vi "NT1-Main.vi"() -> ()   [LabVIEW 2019]
uses:
  Get-Elapsed-Time.vi
  IsError.vi
  <vilib>/Rock Robotics/Network Tables/NT Globals.vi
  <vilib>/Rock Robotics/Network Tables/Manage Connection List.vi
  <vilib>/Rock Robotics/Network Tables/NT Write String Array.vi
  <vilib>/Rock Robotics/Network Tables/NT Write String.vi
  <vilib>/Rock Robotics/Network Tables/NT Write Numeric Array.vi
  <vilib>/Rock Robotics/Network Tables/NT Write Number.vi
  <vilib>/Rock Robotics/Network Tables/NT Write Boolean Array.vi
  <vilib>/Rock Robotics/Network Tables/NT Write Boolean.vi
  <vilib>/Rock Robotics/Network Tables/NT Read Boolean.vi
  <vilib>/Rock Robotics/Network Tables/NT Read Boolean Array.vi
  <vilib>/Rock Robotics/Network Tables/NT Read Number.vi
  <vilib>/Rock Robotics/Network Tables/NT Read Numeric Array.vi
  <vilib>/Rock Robotics/Network Tables/NT Read String.vi
  <vilib>/Rock Robotics/Network Tables/NT Read String Array.vi
  <vilib>/Rock Robotics/WPI/ThirdParty/JAS_Junk/TrajLib/Util_GetTime.vi
  NTJ_OldVer_FlushSingle.vi
  <vilib>/Rock Robotics/Network Tables/NT Flush Data Updates.vi
panel:
  out "Srv Test3 ID":i32 format="%11d"
  out "Srv Test2 ID":i32 format="%11d"
  out "Srv Test1 ID":i32 format="%11d"
  out "Srv Test0  ID":i32 format="%11d"
  out "Srv Test3 Seq":u16 format="0x%04x"
  out "Srv Test2 Seq":u16 format="0x%04x"
  out "Srv Test1 Seq":u16 format="0x%04x"
  out "Srv Test0  Seq":u16 format="0x%04x"
  out "Test3 ID":i32 format="%11d"
  out "Test2 ID":i32 format="%11d"
  out "Test1 ID":i32 format="%11d"
  out "Test0  ID":i32 format="%11d"
  out "Serv Test3":dbl
  out "Serv Test2":dbl
  out "ServTest1":dbl
  out "Serv Test0":dbl
  out "Serv Flush\nTest0":bool=TRUE
  out "Serv Set Fast":bool=TRUE
  out "Serv Create\nNew":bool=TRUE
  out "Serv Many Fast":bool=TRUE
  out "Serv Del New":bool=TRUE
  out "Serv Del All":bool=TRUE
  out "Serv Test1\nPersist":bool=TRUE
  out "Test1 \nPersist (flg)":bool=TRUE
  out "Test3 Seq":u16 format="0x%04x"
  out "Test2 Seq":u16 format="0x%04x"
  out "Test1 Seq":u16 format="0x%04x"
  out "Test0  Seq":u16 format="0x%04x"
  out "Test0 \nFast (flg)":bool=TRUE
  out "Test1 \nPersist (list)":bool=TRUE
  in  "Serv Test1 \nPersist":bool
  in  "Test1 Persist":bool
  in  "Test0Fast":bool
  in  "DeleteNew":bool
  in  "ServFlush":bool
  in  "DeleteAll":bool
  in  "Serv\n Many Ent":bool
  in  "Serv\n Test0 Fast":bool
  in  "Serv Del All":bool
  in  "Serv Del New":bool
  in  "Serv Create \nNew":bool
  in  "Many Entries":bool
  in  "CreateNew":bool
  in  "FlusehTest0":bool
  in  "Tab Control":enum32{"Info", "Test", "Tree", "Trend"}(tab)
  out "Rcv Msg 17 / Sec":dbl format="%24.2f"
  out "Test0 Roundtrip\nAvg Time (sec)":dbl format="%16.3f"
  out "Name":string
  out "Start Time":string
  out "Variable Count":i32
  out "Connection\nCount":i32
  out "IsClient":bool
  out "Produce Read Errors":bool
  out "ValidateTable":bool
  out "ConnectionNames":string[](array[string])
  out "InitComplete":bool[](array[boolean])
  out "Robot CPU Use":dbl format="%16.3f"
  out "Send Msg 17 / Sec":dbl format="%24.2f"
  out "NT Connection":bool
  out "Connection \nCount":i32
  out "StillLooping":i64
  out "Test-String":string
  out "Test-StringArray":string[](array[string])
  out "Test-NumbArray":dbl[](array[numeric])
  out "Test-BoolArray":bool[](array[boolean])
  out "Test-Bool":bool
  out "Test-Numb":dbl
  out "Tree":string(tree)
  in  "Update":enum16{"0.1 Sec", "1 Second", "10 Second"}(ring)=enum."1 Second"
  out "Server Msg 17 Processing (Per / Sec)":T1(graph)
  out "Server CPU Use / 4 Client Round Trip Time":T2(graph)
  out "Good3":bool
  out "Good2":bool
  out "Good1":bool
  out "Good0":bool
  out "Test3":dbl
  out "Test2":dbl
  out "Test1":dbl
  out "Test0":dbl
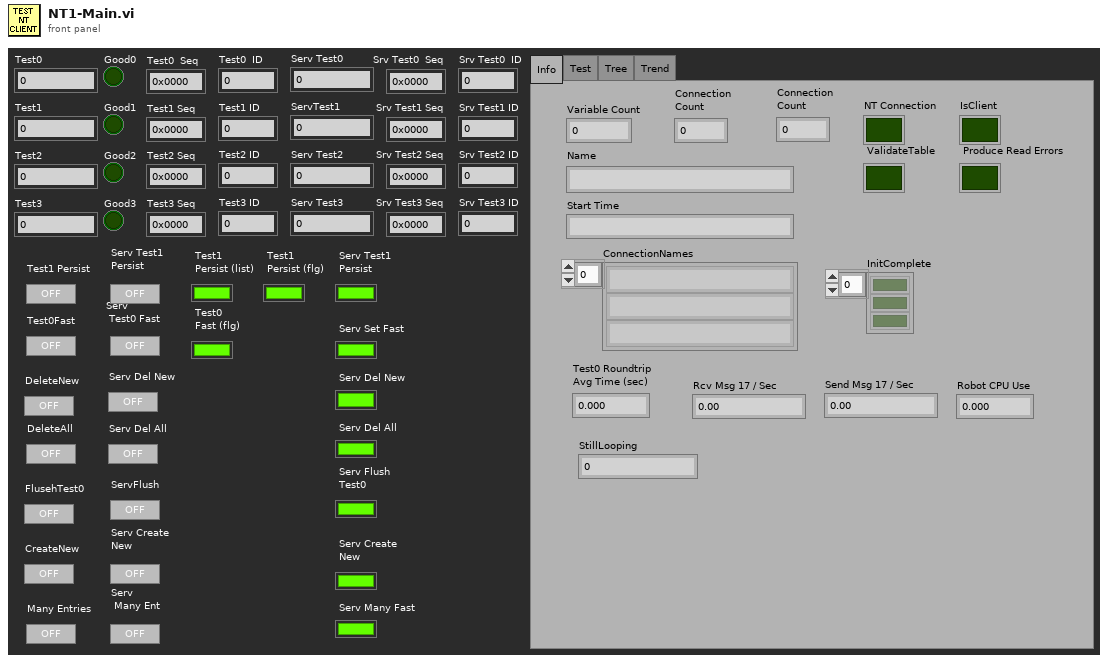
[diagram p1: front panel]
types:
  T1 = cluster{"Rcv Msg 17 / Sec":dbl, "Send Msg 17 / Sec":dbl}
  T2 = cluster{"Robot CPU Use":dbl, "Test0 Roundtrip\nAvg Time (sec)":dbl}
  T3 = cluster{"Shift":bool, "Ctrl":bool, "Alt":bool, "Cmd":bool, "Opt":bool}
  T4 = typedef "Field Data.ctl" = cluster{"Dbl":dbl, "String":string, "Type":T5, "Boolean":bool, "Sequence #":T6, "Flags":u8}
  T5 = typedef "Field Type.ctl" = enum8{"Invalid", "Bool", "Numeric", "String", "Raw", "Boolean Array", "Numeric Array", "String Array", "RPC"}
  T6 = typedef "Sequence.ctl" = u16
  T7 = typedef "Field ID.ctl" = i32
  T8 = typedef "LVDateTimeRec.ctl" = cluster{"fractional second":dbl, "second":i32, "minute":i32, "hour":i32, "day of month":i32, "month":i32, "year":i32, "day of week":i32, "day of year":i32, "DST":i32}
  T9 = typedef "ClientNTTestConfig.ctl" = cluster{"Elapsed0":string, "Name0":string, "Test0":u32, "Ellapsed1":string, "Name1":string, "Test1":u32, "Elapsed2":string, "Name2":string, "Test2":u32, "Elapsed3":string, "Name3":string, "Test3":u32, "NewName":string}
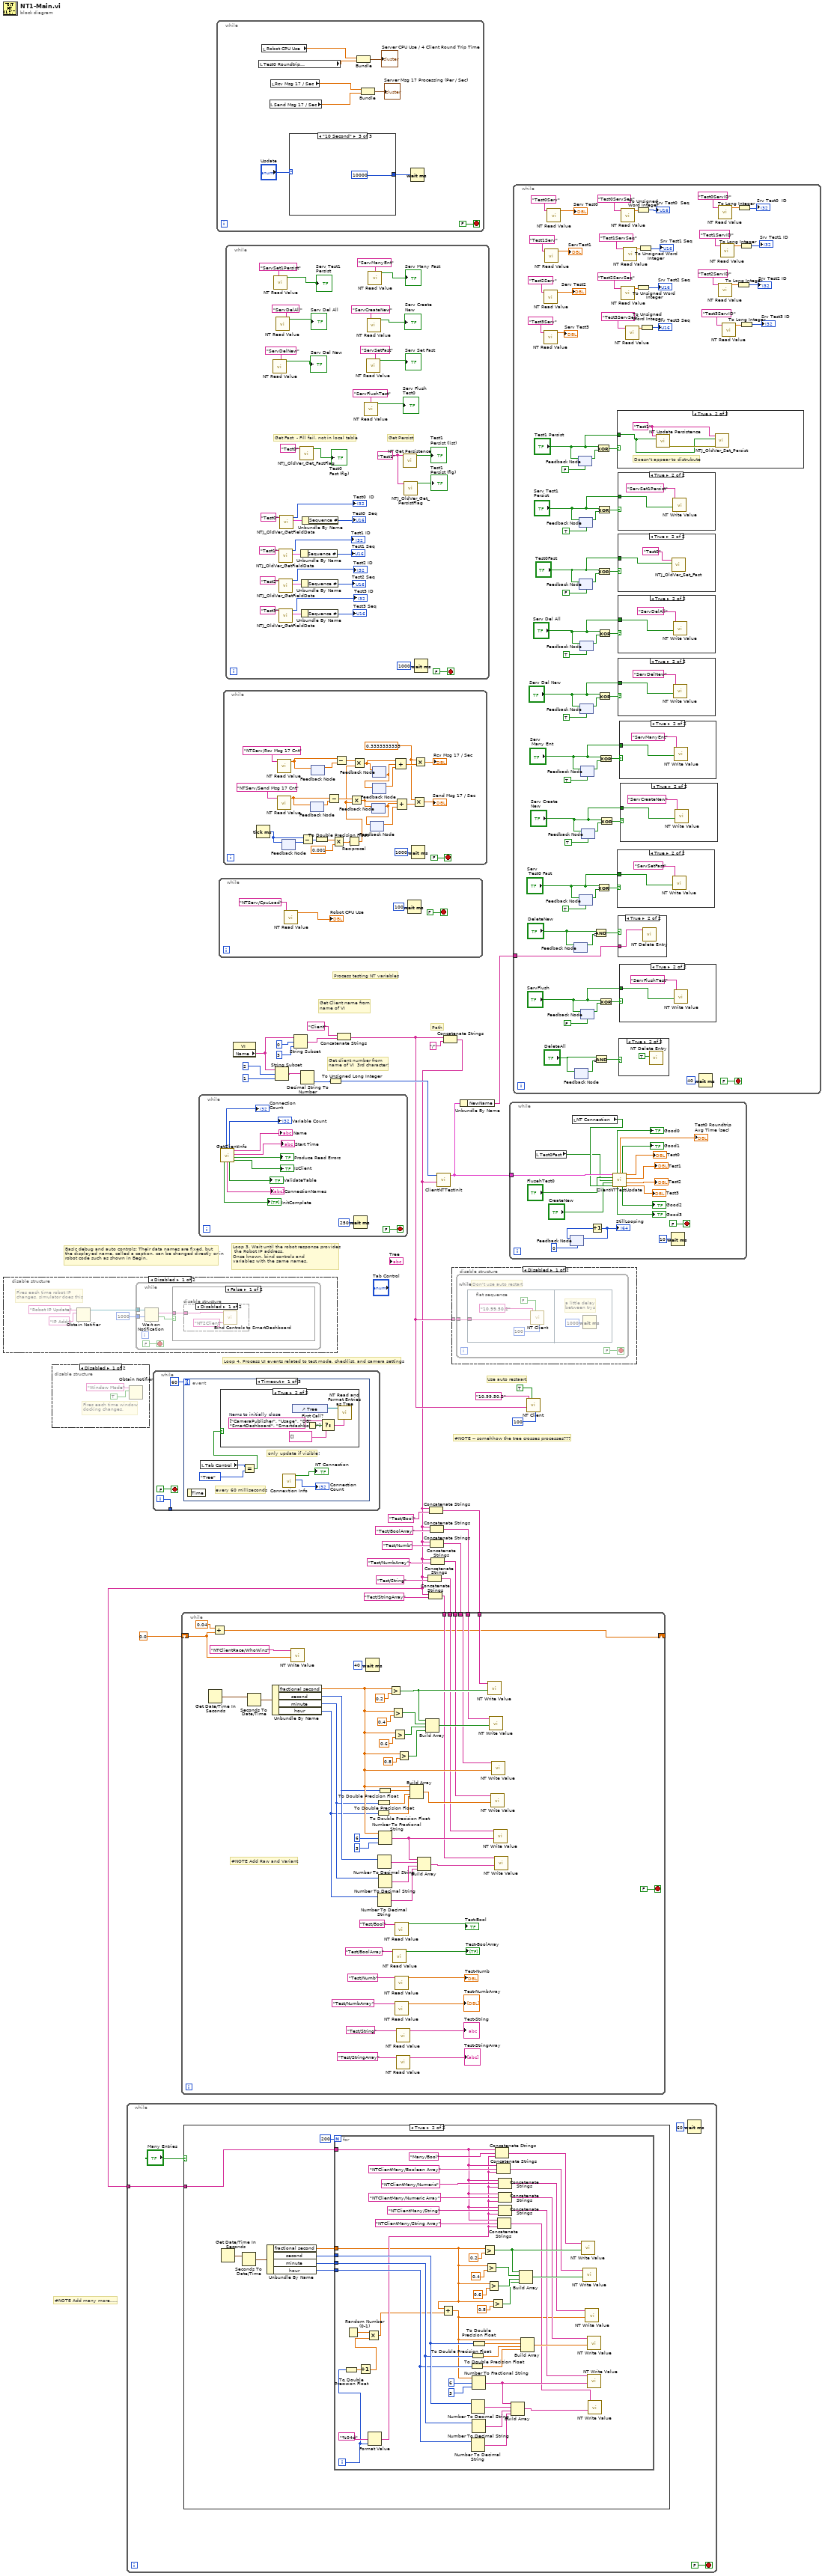
[diagram p0: block diagram]
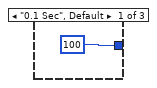
[diagram p2: hidden frame]
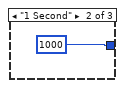
[diagram p3: hidden frame]
diagram:
  # "#NOTE Add many more....."
  # "Path"
  # "Get Client name from\nname of VI"
  # "Get client number from\nname of VI  3rd character!"
  # "Process testing NT variables"
  # "Use auto restaart"
  # "#NOTE -- somehhow the tree crosses processes???"
  # "Basic debug and auto controls: Their data names are fixed, but\nthe displayed name, called a caption, can be changed directly or in\nrobot code such as shown in Begin."
  # "Loop 4. Process UI events related to test mode, checklist, and camera settings"
  # "Loop 3. Wait until the robot response provides\n the Robot IP address.\nOnce known, bind controls and\nvariables with the same names."
  n1 = disable-structure shown="Disabled" {
    frame Disabled {
      # "Fires each time robot IP\nchanges, simulator does this"
      n2 = Obtain Notifier(name (unnamed)="Robot IP Update", notification data type="IP Addr" ("name (unnamed)")) -> (notifier out=w32:refnum<notifier>)  [unwired: 2 in, 2 out]
      n3 = while {
        tunnel: w32 -> [w39]
        tunnel: u32 1000 ("milliseconds to wait") -> [w37]
        stop <- FALSE stop-if-true
        n4 = Wait on Notification(notifier=w39, timeout in ms (-1)=w37) -> (notification=w38:string, timed out?=w36:bool)  [unwired: 2 in, 2 out]
        n5 = case shown="False" w36 {
          tunnel: w38 -> [w41 _]
          frame False {
            n6 = disable-structure shown="Disabled" {
              disable-tunnel: w41 -> [w43 _]
              frame Disabled {
                n7 = call <vilib>:"Bind Controls to SmartDashboard.vi"("Client Name"="NT2Client", "Server IP Address"=w43) -> ()  [unwired: 10 in]
              }
              frame Enabled {
              }
            }
          }
          frame True {
          }
        }
      }
    }
    frame Enabled {
    }
  }
  n8 = disable-structure shown="Disabled" {
    frame Disabled {
      # "Fires each time window\ndocking changes."
      n9 = Obtain Notifier(name (unnamed)="Window Mode", notification data type=TRUE) -> ()  [unwired: 2 in, 3 out]
    }
    frame Enabled {
    }
  }
  n10 = while {
    tunnel: [w46] -> _
    i -> [w46]
    stop <- FALSE stop-if-true
    n11 = event shown="[0] Timeout" {
      selector: _ -> [_ _ _]
      dyn-events: _ -> [_ _ _]
      timeout: u32 60 ("milliseconds to wait") -> [_ _ _]
      event Timeout {
        # "only update if visible!"
        # "every 60 milliseconds"
        n12 = event-data() -> ()  [unwired: 1 in, 1 out]
        n13 = local read "Tab Control"() -> (w51:enum32{"Info", "Test", "Tree", "Trend"})
        n14 = Equal?(x=w51, y=enum32{"Info", "Test", "Tree"}."Tree") -> (x = y?=w50:bool)
        n15 = case shown="True" w50 {
          frame False {
          }
          frame True {
            w58 = string[] ["CameraPublisher", "Usage", "DB", "SmartDashboard", "Smartdashboard"]  # Items to initially close
            n16 = control-ref of="Tree"() -> (w56:refnum<vi>)
            n17 = First Call?() -> (First Call?: T/F=w55:bool)
            n18 = Select(t=w58, s=w55, f=string[] []) -> (s? t:f=w54:string[])
            n19 = call <vilib>:"NT Read and Format Entries as Tree.vi"("Tags to  Close"=w54, "Tree Refnum"=w56) -> ()  [unwired: 8 in, 2 out]
          }
        }
        n20 = call <vilib>:"Connextion Info.vi"() -> ("Connection Count"=→"Connection \nCount":i32, "Connected"=→"NT Connection":bool)  [unwired: 10 in]
      }
      event Panel Close {
        n21 = event-data() -> ()  [unwired: 1 in, 1 out]
        n22 = invoke class="VI" method="Abort VI"() -> ()  [unwired: 3 in, 3 out]
      }
      event "Tree": Double Click {
        # "Update variable's persistence setting,\nif it is a true variable and not a category"
        n23 = event-data() -> ("PlatMods"=w60:T3, "Tag"=w59:string)  [unwired: 1 in]
        n24 = Unbundle(w60) -> ("Shift"=w64:bool)  [unwired: 4 out]
        n25 = String Subset(string=w59, length (rest)=1 ("length (rest)")) -> (substring=w61:string)  [unwired: 1 in]
        n26 = Not(x=w64) -> (.not. x?=w63:bool)
        n27 = case shown="\"/\"" w61 {
          tunnel: w63 -> [_ w66]
          tunnel: w59 -> [_ w65]
          frame Default {
          }
          frame "/" {
            n28 = call <vilib>:"NT Update Persistence.vi"("Persistence"=w66, "Name"=w65) -> ()  [unwired: 9 in, 1 out]
          }
        }
      }
    }
  }
  n29 = while {
    stop <- FALSE stop-if-true
    n30 = call "GetClientInfo.vi"() -> ("IsClient"=→"IsClient":bool, "Produce Read Errors"=→"Produce Read Errors":bool, "Start Time"=→"Start Time":string, "Name"=→"Name":string, "ValidateTable"=→"ValidateTable":bool, "Variable Count"=→"Variable Count":i32, "ConnectionNames"=→"ConnectionNames":string[], "ConnectionCount"=→"Connection\nCount":i32, "InitComplete"=→"InitComplete":bool[])  [unwired: 3 in]
    n31 = Wait (ms)(milliseconds to wait=u32 250) -> ()  [unwired: 1 out]
  }
  n32 = while {
    stop <- FALSE stop-if-true
    n33 = local read "Test0 Roundtrip\nAvg Time (sec)"() -> (w79:dbl)
    n34 = local read "Robot CPU Use"() -> (w80:dbl)
    n35 = local read "Send Msg 17 / Sec"() -> (w83:dbl)
    n36 = local read "Rcv Msg 17 / Sec"() -> (w84:dbl)
    n37 = case shown="\"10 Second\"" "Update" {
      tunnel: [u32 100 ("milliseconds to wait") u32 1000 ("milliseconds to wait") u32 10000 ("milliseconds to wait")] -> w85
      frame "0.1 Sec", Default {
      }
      frame "1 Second" {
      }
      frame "10 Second" {
      }
    }
    n38 = Bundle("Robot CPU Use"=w80, "Test0 Roundtrip\nAvg Time (sec)"=w79) -> (→"Server CPU Use / 4 Client Round Trip Time":T2)  [unwired: 1 in]
    n39 = Bundle("Rcv Msg 17 / Sec"=w84, "Send Msg 17 / Sec"=w83) -> (→"Server Msg 17 Processing (Per / Sec)":T1)  [unwired: 1 in]
    n40 = Wait (ms)(milliseconds to wait=w85) -> ()  [unwired: 1 out]
  }
  n41 = while {
    stop <- FALSE stop-if-true
    n42 = call-poly <vilib>:"NT Read Value.vi"("Name"="NTServ/CpuLoad") -> ("Numeric"=→"Robot CPU Use":dbl)  [unwired: 9 in, 1 out]
    n43 = Wait (ms)(milliseconds to wait=u32 100) -> ()  [unwired: 1 out]
  }
  n44 = while {
    stop <- FALSE stop-if-true
    w101 = 0.3333333333 ("x")
    n45 = Tick Count (ms)() -> (millisecond timer value=w103:u32)
    n46 = call-poly <vilib>:"NT Read Value.vi"("Name"="NTServ/Send Msg 17 Cnt") -> ("Numeric"=w118:dbl)  [unwired: 9 in, 1 out]
    n47 = call-poly <vilib>:"NT Read Value.vi"("Name"="NTServ/Rcv Msg 17 Cnt") -> ("Numeric"=w115:dbl)  [unwired: 9 in, 1 out]
    n48 = feedback #1() -> (w102:u32)  [unwired: 1 in]
    n49 = feedback-in #1(w103) -> ()
    n50 = Subtract(x=w103, y=w102) -> (x-y=w104:u32)
    n51 = feedback #2() -> (w119:dbl)  [unwired: 1 in]
    n52 = feedback-in #2(w118) -> ()
    n53 = feedback #3() -> (w116:dbl)  [unwired: 1 in]
    n54 = feedback-in #3(w115) -> ()
    n55 = To Double Precision Float(number=w104) -> (double precision float=w105:dbl)
    n56 = Subtract(x=w118, y=w119) -> (x-y=w117:dbl)
    n57 = Multiply(x=w105, y=0.001) -> (x*y=w106:dbl)
    n58 = Subtract(x=w115, y=w116) -> (x-y=w114:dbl)
    n59 = Reciprocal(x=w106) -> (1/x=w107:dbl)
    n60 = Multiply(x=w117, y=w107) -> (x*y=w111:dbl)
    n61 = Multiply(x=w114, y=w107) -> (x*y=w108:dbl)
    n62 = feedback #4() -> (w94:dbl)  [unwired: 1 in]
    n63 = feedback #5() -> (w95:dbl)  [unwired: 1 in]
    n64 = feedback-in #4(w95) -> ()
    n65 = feedback-in #5(w111) -> ()
    n66 = feedback #6() -> (w96:dbl)  [unwired: 1 in]
    n67 = feedback #7() -> (w97:dbl)  [unwired: 1 in]
    n68 = feedback-in #6(w97) -> ()
    n69 = feedback-in #7(w108) -> ()
    n70 = Compound Arithmetic op=ADD(w108, w97, w96) -> (w109:dbl)
    n71 = Compound Arithmetic op=ADD(w111, w95, w94) -> (w110:dbl)
    n72 = Wait (ms)(milliseconds to wait=u32 1000) -> ()  [unwired: 1 out]
    n73 = Multiply(x=w101, y=w110) -> (x*y=→"Send Msg 17 / Sec":dbl)
    n74 = Multiply(x=w101, y=w109) -> (x*y=→"Rcv Msg 17 / Sec":dbl)
  }
  n75 = while {
    stop <- FALSE stop-if-true
    w123 = "Test1" ("Name")
    # "Get Persist"
    # "Get Fast  - Fill fail, not in local table"
    n76 = call-poly <vilib>:"NT Read Value.vi"("Name"="ServDelNew") -> ("Boolean"=→"Serv Del New":bool)  [unwired: 9 in, 1 out]
    n77 = call-poly <vilib>:"NT Read Value.vi"("Name"="ServSet1Persist") -> ("Boolean"=→"Serv Test1\nPersist":bool)  [unwired: 9 in, 1 out]
    n78 = call-poly <vilib>:"NT Read Value.vi"("Name"="ServDelAll") -> ("Boolean"=→"Serv Del All":bool)  [unwired: 9 in, 1 out]
    n79 = call "NTJ_OldVer_GetFieldData.vi"("Entry Name"="Test1") -> ("Field Value Out"=w149:T4, "Entry ID"=→"Test1 ID":T7)  [unwired: 7 in, 1 out]
    n80 = call "NTJ_OldVer_GetFieldData.vi"("Entry Name"="Test2") -> ("Field Value Out"=w147:T4, "Entry ID"=→"Test2 ID":T7)  [unwired: 7 in, 1 out]
    n81 = call "NTJ_OldVer_GetFieldData.vi"("Entry Name"="Test3") -> ("Field Value Out"=w145:T4, "Entry ID"=→"Test3 ID":T7)  [unwired: 7 in, 1 out]
    n82 = call "NTJ_OldVer_GetFieldData.vi"("Entry Name"="Test0") -> ("Field Value Out"=w152:T4, "Entry ID"=→"Test0  ID":T7)  [unwired: 7 in, 1 out]
    n83 = call "NTJ_OldVer_Get_FastFlag.vi"("Entry Name"="Test0") -> ("FastFlag"=→"Test0 \nFast (flg)":bool)  [unwired: 9 in, 1 out]
    n84 = Unbundle By Name(w149) -> ("Sequence #"=→"Test1 Seq":T6)
    n85 = Unbundle By Name(w147) -> ("Sequence #"=→"Test2 Seq":T6)
    n86 = Unbundle By Name(w145) -> ("Sequence #"=→"Test3 Seq":T6)
    n87 = Unbundle By Name(w152) -> ("Sequence #"=→"Test0  Seq":T6)
    n88 = call-poly <vilib>:"NT Read Value.vi"("Name"="ServFlushTest") -> ("Boolean"=→"Serv Flush\nTest0":bool)  [unwired: 9 in, 1 out]
    n89 = call-poly <vilib>:"NT Read Value.vi"("Name"="ServSetFast") -> ("Boolean"=→"Serv Set Fast":bool)  [unwired: 9 in, 1 out]
    n90 = call-poly <vilib>:"NT Read Value.vi"("Name"="ServCreateNew") -> ("Boolean"=→"Serv Create\nNew":bool)  [unwired: 9 in, 1 out]
    n91 = call-poly <vilib>:"NT Read Value.vi"("Name"="ServManyEnt") -> ("Boolean"=→"Serv Many Fast":bool)  [unwired: 9 in, 1 out]
    n92 = call <vilib>:"NT Get Persistence.vi"("Name"=w123) -> ("Persistence"=→"Test1 \nPersist (list)":bool)  [unwired: 9 in, 1 out]
    n93 = call "NTJ_OldVer_Get_PersistFlag.vi"("Entry Name"=w123) -> ("PersistFlag"=→"Test1 \nPersist (flg)":bool)  [unwired: 9 in, 1 out]
    n94 = Wait (ms)(milliseconds to wait=u32 1000) -> ()  [unwired: 1 out]
  }
  n95 = property class="VI"() -> ("Name"=w22:string)  [unwired: 2 in, 2 out]
  n96 = String Subset(string=w22, offset (0)=2, length (rest)=1 ("length (rest)")) -> (substring=w26:string)
  n97 = String Subset(string=w22, offset (0)=0, length (rest)=3 ("length (rest)")) -> (substring=w19:string)
  n98 = Decimal String To Number(string=w26) -> (number=w25:i32)  [unwired: 2 in, 1 out]
  n99 = To Unsigned Long Integer(number=w25) -> (unsigned 32bit integer=w24:u32)
  n100 = Concatenate Strings("Client" ("string"), w19) -> (w17:string)
  n101 = Concatenate Strings(w17, "/" ("string")) -> (w1:string)
  n102 = while {
    tunnel: w1 -> [w159]
    stop <- FALSE stop-if-true
    n103 = case shown="True" "Many Entries" {
      tunnel: w159 -> [_ w164]
      frame False {
      }
      frame True {
        n104 = Get Date/Time In Seconds() -> (seconds since 1Jan1904=w170:timestamp)
        n105 = Seconds To Date/Time(time stamp (now)=w170) -> (date time rec=w169:T8)  [unwired: 1 in]
        n106 = Unbundle By Name(w169) -> ("fractional second"=w168:dbl, "second"=w167:i32, "minute"=w166:i32, "hour"=w165:i32)
        n107 = for {
          N: 200 -> [_]
          tunnel: w168 -> [w172]
          tunnel: w167 -> [w199]
          tunnel: w166 -> [w198]
          tunnel: w165 -> [w197]
          tunnel: w164 -> [w186]
          i -> [w175]
          n108 = To Double Precision Float(number=w175) -> (double precision float=w176:dbl)
          n109 = Random Number (0-1)() -> (number: 0 to 1=w177:dbl)
          n110 = Increment(x=w176) -> (x+1=w174:dbl)
          n111 = Multiply(x=w177, y=w174) -> (x*y=w171:dbl)
          n112 = Format Value(format string="%04d", value (0)=w175) -> (output string=w178:string)  [unwired: 1 in]
          n113 = Add(x=w172, y=w171) -> (x+y=w173:dbl)
          n114 = To Double Precision Float(number=w197) -> (double precision float=w204:dbl)
          n115 = To Double Precision Float(number=w198) -> (double precision float=w205:dbl)
          n116 = Number To Decimal String(number=w197) -> (decimal integer string=w194:string)  [unwired: 1 in]
          n117 = Number To Decimal String(number=w199) -> (decimal integer string=w196:string)  [unwired: 1 in]
          n118 = Number To Fractional String(number=w173, width (-)=i16 6, precision (6)=i16 3) -> (F-format string=w200:string)  [unwired: 1 in]
          n119 = Number To Decimal String(number=w198) -> (decimal integer string=w195:string)  [unwired: 1 in]
          n120 = To Double Precision Float(number=w199) -> (double precision float=w206:dbl)
          n121 = Greater?(x=w172, y=0.2) -> (0:w211:bool)
          n122 = Greater?(x=w172, y=0.4) -> (0:w210:bool)
          n123 = Greater?(x=w172, y=0.6) -> (0:w209:bool)
          n124 = Greater?(x=w172, y=0.8) -> (0:w208:bool)
          n125 = Concatenate Strings(w186, "Many/Bool" ("Name"), w178) -> (w185:string)
          n126 = Concatenate Strings(w186, "NTClientMany/Boolean Array" ("Name"), w178) -> (w184:string)
          n127 = Concatenate Strings(w186, "NTClientMany/String Array" ("Name"), w178) -> (w180:string)
          n128 = Concatenate Strings(w186, "NTClientMany/Numeric" ("Name"), w178) -> (w183:string)
          n129 = Concatenate Strings(w186, "NTClientMany/Numeric Array" ("Name"), w178) -> (w182:string)
          n130 = Concatenate Strings(w186, "NTClientMany/String" ("Name"), w178) -> (w181:string)
          n131 = Build Array(w200, w196, w195, w194) -> (w193:string[])
          n132 = Build Array(w211, w210, w209, w208) -> (w207:bool[])
          n133 = Build Array(w173, w206, w205, w204) -> (w203:dbl[])
          n134 = call-poly <vilib>:"NT Write Value.vi"("Boolean"=w211, "Name"=w185) -> ()  [unwired: 9 in, 1 out]
          n135 = call-poly <vilib>:"NT Write Value.vi"("Boolean Array"=w207, "Name"=w184) -> ()  [unwired: 9 in, 1 out]
          n136 = call-poly <vilib>:"NT Write Value.vi"("Numeric"=w173, "Name"=w183) -> ()  [unwired: 9 in, 1 out]
          n137 = call-poly <vilib>:"NT Write Value.vi"("Numeric Array"=w203, "Name"=w182) -> ()  [unwired: 9 in, 1 out]
          n138 = call-poly <vilib>:"NT Write Value.vi"("String"=w200, "Name"=w181) -> ()  [unwired: 9 in, 1 out]
          n139 = call-poly <vilib>:"NT Write Value.vi"("String Array"=w193, "Name"=w180) -> ()  [unwired: 9 in, 1 out]
        }
      }
    }
    n140 = Wait (ms)(milliseconds to wait=u32 60) -> ()  [unwired: 1 out]
  }
  n141 = Concatenate Strings(w1, "Test/String" ("Name")) -> (w6:string)
  n142 = Concatenate Strings(w1, "Test/StringArray" ("Name")) -> (w4:string)
  n143 = Concatenate Strings(w1, "Test/Bool" ("Name")) -> (w14:string)
  n144 = Concatenate Strings(w1, "Test/BoolArray" ("Name")) -> (w12:string)
  n145 = Concatenate Strings(w1, "Test/Numb" ("Name")) -> (w10:string)
  n146 = Concatenate Strings(w1, "Test/NumbArray" ("Name")) -> (w8:string)
  n147 = while {
    tunnel: w14 -> [w237]
    tunnel: w12 -> [w236]
    tunnel: w10 -> [w235]
    tunnel: w8 -> [w234]
    tunnel: w6 -> [w233]
    tunnel: w4 -> [w232]
    shift-right: [w216] -> _
    shift-left: 0.0 -> [w218]
    stop <- FALSE stop-if-true
    # "#NOTE Add Raw and Variant"
    n148 = Get Date/Time In Seconds() -> (seconds since 1Jan1904=w265:timestamp)
    n149 = Add(x=0.04, y=w218) -> (x+y=w216:dbl)
    n150 = Seconds To Date/Time(time stamp (now)=w265) -> (date time rec=w264:T8)  [unwired: 1 in]
    n151 = Unbundle By Name(w264) -> ("fractional second"=w248:dbl, "second"=w244:i32, "minute"=w243:i32, "hour"=w242:i32)
    n152 = call-poly <vilib>:"NT Write Value.vi"("Numeric"=w218, "Name"="NTClientRace/WhoWins") -> ()  [unwired: 9 in, 1 out]
    n153 = Wait (ms)(milliseconds to wait=u32 40) -> ()  [unwired: 1 out]
    n154 = To Double Precision Float(number=w242) -> (double precision float=w250:dbl)
    n155 = To Double Precision Float(number=w243) -> (double precision float=w251:dbl)
    n156 = Number To Decimal String(number=w242) -> (decimal integer string=w239:string)  [unwired: 1 in]
    n157 = Number To Decimal String(number=w244) -> (decimal integer string=w241:string)  [unwired: 1 in]
    n158 = Number To Fractional String(number=w248, width (-)=i16 6, precision (6)=i16 3) -> (F-format string=w245:string)  [unwired: 1 in]
    n159 = Number To Decimal String(number=w243) -> (decimal integer string=w240:string)  [unwired: 1 in]
    n160 = To Double Precision Float(number=w244) -> (double precision float=w252:dbl)
    n161 = Greater?(x=w248, y=0.2) -> (0:w259:bool)
    n162 = Greater?(x=w248, y=0.4) -> (0:w258:bool)
    n163 = call-poly <vilib>:"NT Read Value.vi"("Name"="Test/BoolArray") -> ("Boolean Array"=→"Test-BoolArray":bool[])  [unwired: 9 in, 1 out]
    n164 = Greater?(x=w248, y=0.6) -> (0:w257:bool)
    n165 = call-poly <vilib>:"NT Read Value.vi"("Name"="Test/Bool") -> ("Boolean"=→"Test-Bool":bool)  [unwired: 9 in, 1 out]
    n166 = call-poly <vilib>:"NT Read Value.vi"("Name"="Test/Numb") -> ("Numeric"=→"Test-Numb":dbl)  [unwired: 9 in, 1 out]
    n167 = call-poly <vilib>:"NT Read Value.vi"("Name"="Test/NumbArray") -> ("Numeric Array"=→"Test-NumbArray":dbl[])  [unwired: 9 in, 1 out]
    n168 = call-poly <vilib>:"NT Read Value.vi"("Name"="Test/String") -> ("String"=→"Test-String":string)  [unwired: 9 in, 1 out]
    n169 = call-poly <vilib>:"NT Read Value.vi"("Name"="Test/StringArray") -> ("String Array"=→"Test-StringArray":string[])  [unwired: 9 in, 1 out]
    n170 = Greater?(x=w248, y=0.8) -> (0:w256:bool)
    n171 = Build Array(w248, w252, w251, w250) -> (w249:dbl[])
    n172 = Build Array(w245, w241, w240, w239) -> (w238:string[])
    n173 = Build Array(w259, w258, w257, w256) -> (w253:bool[])
    n174 = call-poly <vilib>:"NT Write Value.vi"("Boolean"=w259, "Name"=w237) -> ()  [unwired: 9 in, 1 out]
    n175 = call-poly <vilib>:"NT Write Value.vi"("Boolean Array"=w253, "Name"=w236) -> ()  [unwired: 9 in, 1 out]
    n176 = call-poly <vilib>:"NT Write Value.vi"("Numeric Array"=w249, "Name"=w234) -> ()  [unwired: 9 in, 1 out]
    n177 = call-poly <vilib>:"NT Write Value.vi"("Numeric"=w248, "Name"=w235) -> ()  [unwired: 9 in, 1 out]
    n178 = call-poly <vilib>:"NT Write Value.vi"("String"=w245, "Name"=w233) -> ()  [unwired: 9 in, 1 out]
    n179 = call-poly <vilib>:"NT Write Value.vi"("String Array"=w238, "Name"=w232) -> ()  [unwired: 9 in, 1 out]
  }
  n180 = call "ClientNTTestInit.vi"("Prefix"=w1, "Instance"=w24) -> ("TestConfig"=w18:T9)  [unwired: 9 in]
  n181 = disable-structure shown="Disabled" {
    disable-tunnel: w17 -> [w266 _]
    frame Disabled {
      n182 = while {
        tunnel: w266 -> [w267]
        stop <- FALSE stop-if-true
        # "Don't use auto restart"
        n183 = flat-sequence {
          tunnel: w267 -> [w269]
          frame #0 {
            n184 = call <vilib>:"NT Client.vi"("Update Time"=100, "Automatic restart"=FALSE, "Client Name"=w269, "Server IP Address"="10.99.50.2") -> ()  [unwired: 8 in]
          }
          frame #1 {
            # "a little delay\nbetween trys"
            n185 = Wait (ms)(milliseconds to wait=u32 1000) -> ()  [unwired: 1 out]
          }
        }
      }
    }
    frame Enabled {
    }
  }
  n186 = Unbundle By Name(w18) -> ("NewName"=w2:string)
  n187 = while {
    tunnel: w18 -> [w292]
    stop <- FALSE stop-if-true
    n188 = local read "Test0Fast"() -> (w274:bool)
    n189 = feedback #8(i64 0) -> (w275:i64)
    n190 = local read "NT Connection"() -> (w281:bool)
    n191 = Increment(x=w275) -> (x+1=w277:i64)
    "StillLooping" <- w277
    n192 = feedback-in #8(w277) -> ()
    n193 = call "ClientNTTestUpdate.vi"("TestConfig"=w292, "Flush0"="FlusehTest0", "SimulateFast0"=w274, "CreateTestNew"="CreateNew", "NT Connection"=w281) -> ("Good0"=→"Good0":bool, "Test0RoundTripTime"=→"Test0 Roundtrip\nAvg Time (sec)":dbl, "Good1"=→"Good1":bool, "Value0"=→"Test0":dbl, "Value1"=→"Test1":dbl, "Value2"=→"Test2":dbl, "Good3"=→"Good3":bool, "Good2"=→"Good2":bool, "Value3"=→"Test3":dbl)  [unwired: 2 in]
    n194 = Wait (ms)(milliseconds to wait=u32 10) -> ()  [unwired: 1 out]
  }
  n195 = while {
    tunnel: w2 -> [w357]
    stop <- FALSE stop-if-true
    n196 = call-poly <vilib>:"NT Read Value.vi"("Name"="Test3Serv") -> ("Numeric"=→"Serv Test3":dbl)  [unwired: 9 in, 1 out]
    n197 = call-poly <vilib>:"NT Read Value.vi"("Name"="Test2Serv") -> ("Numeric"=→"Serv Test2":dbl)  [unwired: 9 in, 1 out]
    n198 = call-poly <vilib>:"NT Read Value.vi"("Name"="Test1Serv") -> ("Numeric"=→"ServTest1":dbl)  [unwired: 9 in, 1 out]
    n199 = call-poly <vilib>:"NT Read Value.vi"("Name"="Test0Serv") -> ("Numeric"=→"Serv Test0":dbl)  [unwired: 9 in, 1 out]
    n200 = feedback #9() -> (w360:bool)  [unwired: 1 in]
    n201 = feedback-in #9("DeleteNew") -> ()
    n202 = feedback #10() -> (w366:bool)  [unwired: 1 in]
    n203 = feedback-in #10("DeleteAll") -> ()
    n204 = feedback #11(FALSE ("ServFlush")) -> (w329:bool)
    n205 = feedback-in #11("Test1 Persist") -> ()
    n206 = feedback #12(TRUE ("ServFlush")) -> (w355:bool)
    n207 = feedback-in #12("Serv\n Test0 Fast") -> ()
    n208 = feedback #13(TRUE ("ServFlush")) -> (w332:bool)
    n209 = feedback-in #13("Serv Test1 \nPersist") -> ()
    n210 = feedback #14(FALSE ("ServFlush")) -> (w335:bool)
    n211 = feedback-in #14("Test0Fast") -> ()
    n212 = feedback #15(TRUE ("ServFlush")) -> (w342:bool)
    n213 = feedback-in #15("Serv Del All") -> ()
    n214 = feedback #16(TRUE ("ServFlush")) -> (w345:bool)
    n215 = feedback-in #16("Serv Del New") -> ()
    n216 = feedback #17(TRUE ("ServFlush")) -> (w348:bool)
    n217 = feedback-in #17("Serv\n Many Ent") -> ()
    n218 = feedback #18(FALSE ("ServFlush")) -> (w363:bool)
    n219 = feedback-in #18("ServFlush") -> ()
    n220 = feedback #19(TRUE ("ServFlush")) -> (w351:bool)
    n221 = feedback-in #19("Serv Create \nNew") -> ()
    n222 = Compound Arithmetic op=AND("DeleteNew", invert w360) -> (w358:bool)
    n223 = Compound Arithmetic op=AND("DeleteAll", invert w366) -> (w367:bool)
    n224 = Exclusive Or(1:w329, 2:"Test1 Persist") -> (0:w328:bool)
    n225 = Exclusive Or(1:w355, 2:"Serv\n Test0 Fast") -> (0:w354:bool)
    n226 = Exclusive Or(1:w332, 2:"Serv Test1 \nPersist") -> (0:w331:bool)
    n227 = Exclusive Or(1:w335, 2:"Test0Fast") -> (0:w334:bool)
    n228 = Exclusive Or(1:w342, 2:"Serv Del All") -> (0:w341:bool)
    n229 = Exclusive Or(1:w345, 2:"Serv Del New") -> (0:w344:bool)
    n230 = Exclusive Or(1:w348, 2:"Serv\n Many Ent") -> (0:w347:bool)
    n231 = Exclusive Or(1:w363, 2:"ServFlush") -> (0:w362:bool)
    n232 = Exclusive Or(1:w351, 2:"Serv Create \nNew") -> (0:w350:bool)
    n233 = case shown="True" w328 {
      tunnel: "Test1 Persist" -> [_ w370]
      frame False {
      }
      frame True {
        w371 = "Test1" ("Name")
        # "Doesn't appear to distrubute"
        n234 = call <vilib>:"NT Update Persistence.vi"("Persistence"=w370, "Name"=w371) -> ("error out"=w372:errorcluster)  [unwired: 9 in]
        n235 = call "NTJ_OldVer_Set_Persist.vi"("error in (no error)"=w372, "Persist Value"=w370, "Entry Name"=w371) -> ()  [unwired: 8 in, 1 out]
      }
    }
    n236 = case shown="True" w354 {
      tunnel: "Serv\n Test0 Fast" -> [_ w385]
      frame False {
      }
      frame True {
        n237 = call-poly <vilib>:"NT Write Value.vi"("Boolean"=w385, "Name"="ServSetFast") -> ()  [unwired: 9 in, 1 out]
      }
    }
    n238 = case shown="True" w331 {
      tunnel: "Serv Test1 \nPersist" -> [_ w373]
      frame False {
      }
      frame True {
        n239 = call-poly <vilib>:"NT Write Value.vi"("Boolean"=w373, "Name"="ServSet1Persist") -> ()  [unwired: 9 in, 1 out]
      }
    }
    n240 = case shown="True" w334 {
      tunnel: "Test0Fast" -> [_ w375]
      frame False {
      }
      frame True {
        n241 = call "NTJ_OldVer_Set_Fast.vi"("Fast Value"=w375, "Entry Name"="Test0") -> ()  [unwired: 9 in, 1 out]
      }
    }
    n242 = case shown="True" w358 {
      tunnel: w357 -> [_ w387]
      frame False {
      }
      frame True {
        n243 = call <vilib>:"NT Delete Entry.vi"("Name"=w387) -> ()  [unwired: 10 in, 1 out]
      }
    }
    n244 = case shown="True" w341 {
      tunnel: "Serv Del All" -> [_ w377]
      frame False {
      }
      frame True {
        n245 = call-poly <vilib>:"NT Write Value.vi"("Boolean"=w377, "Name"="ServDelAll") -> ()  [unwired: 9 in, 1 out]
      }
    }
    n246 = case shown="True" w344 {
      tunnel: "Serv Del New" -> [_ w379]
      frame False {
      }
      frame True {
        n247 = call-poly <vilib>:"NT Write Value.vi"("Boolean"=w379, "Name"="ServDelNew") -> ()  [unwired: 9 in, 1 out]
      }
    }
    n248 = case shown="True" w367 {
      frame False {
      }
      frame True {
        n249 = call <vilib>:"NT Delete Entry.vi"("All"=TRUE) -> ()  [unwired: 10 in, 1 out]
      }
    }
    n250 = case shown="True" w347 {
      tunnel: "Serv\n Many Ent" -> [_ w381]
      frame False {
      }
      frame True {
        n251 = call-poly <vilib>:"NT Write Value.vi"("Boolean"=w381, "Name"="ServManyEnt") -> ()  [unwired: 9 in, 1 out]
      }
    }
    n252 = case shown="True" w362 {
      tunnel: "ServFlush" -> [_ w388]
      frame False {
      }
      frame True {
        n253 = call-poly <vilib>:"NT Write Value.vi"("Boolean"=w388, "Name"="ServFlushTest") -> ()  [unwired: 9 in, 1 out]
      }
    }
    n254 = case shown="True" w350 {
      tunnel: "Serv Create \nNew" -> [_ w383]
      frame False {
      }
      frame True {
        n255 = call-poly <vilib>:"NT Write Value.vi"("Boolean"=w383, "Name"="ServCreateNew") -> ()  [unwired: 9 in, 1 out]
      }
    }
    n256 = call-poly <vilib>:"NT Read Value.vi"("Name"="Test0ServSeq") -> ("Numeric"=w315:dbl)  [unwired: 9 in, 1 out]
    n257 = call-poly <vilib>:"NT Read Value.vi"("Name"="Test2ServSeq") -> ("Numeric"=w310:dbl)  [unwired: 9 in, 1 out]
    n258 = call-poly <vilib>:"NT Read Value.vi"("Name"="Test1ServSeq") -> ("Numeric"=w312:dbl)  [unwired: 9 in, 1 out]
    n259 = call-poly <vilib>:"NT Read Value.vi"("Name"="Test3ServSeq") -> ("Numeric"=w308:dbl)  [unwired: 9 in, 1 out]
    n260 = To Unsigned Word Integer(number=w315) -> (unsigned 16bit integer=→"Srv Test0  Seq":u16)
    n261 = To Unsigned Word Integer(number=w310) -> (unsigned 16bit integer=→"Srv Test2 Seq":u16)
    n262 = To Unsigned Word Integer(number=w312) -> (unsigned 16bit integer=→"Srv Test1 Seq":u16)
    n263 = To Unsigned Word Integer(number=w308) -> (unsigned 16bit integer=→"Srv Test3 Seq":u16)
    n264 = Wait (ms)(milliseconds to wait=u32 40) -> ()  [unwired: 1 out]
    n265 = call-poly <vilib>:"NT Read Value.vi"("Name"="Test0ServID") -> ("Numeric"=w300:dbl)  [unwired: 9 in, 1 out]
    n266 = call-poly <vilib>:"NT Read Value.vi"("Name"="Test2ServID") -> ("Numeric"=w298:dbl)  [unwired: 9 in, 1 out]
    n267 = call-poly <vilib>:"NT Read Value.vi"("Name"="Test1ServID") -> ("Numeric"=w299:dbl)  [unwired: 9 in, 1 out]
    n268 = call-poly <vilib>:"NT Read Value.vi"("Name"="Test3ServID") -> ("Numeric"=w297:dbl)  [unwired: 9 in, 1 out]
    n269 = To Long Integer(number=w298) -> (32bit integer=→"Srv Test2 ID":i32)
    n270 = To Long Integer(number=w300) -> (32bit integer=→"Srv Test0  ID":i32)
    n271 = To Long Integer(number=w299) -> (32bit integer=→"Srv Test1 ID":i32)
    n272 = To Long Integer(number=w297) -> (32bit integer=→"Srv Test3 ID":i32)
  }
  n273 = call <vilib>:"NT Client.vi"("Update Time"=100, "Automatic restart"=TRUE, "Client Name"=w17, "Server IP Address"="10.99.50.2") -> ()  [unwired: 8 in]
